vi "MandelPoint to Pixel.vi"() -> ()   [LabVIEW 2016]
uses:
  MandelPoint.ctl
panel:
  in  "MandelPoint":T1
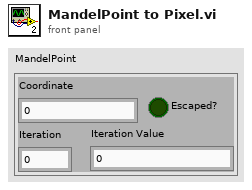
[diagram p1: front panel]
types:
  T1 = typedef "MandelPoint.ctl" = cluster{"Coordinate":cdb, "Iteration":u16, "Escaped? ":bool, "Iteration Value":cdb}
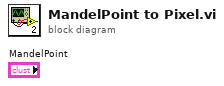
[diagram p0: block diagram]
diagram:
